vi "create_scan_file.vi"(3 "Scan Type":string(combo)="New Scan", 4 "Scan Name":string, 5 "Scan Directory":string="Peter_ferguson\\test_scans\\Tcal Labview\\") -> (0 "Path Scan":path, 1 "Error Out":errorcluster, 2 "Path Spec":path)   [LabVIEW 2020]
uses:
  <vilib>/Utility/sysdir.llb/System Directory Type.ctl
panel:
  out "output string":string
  in  "Leave File Open (T)":bool=TRUE
  out "Report File Name":path
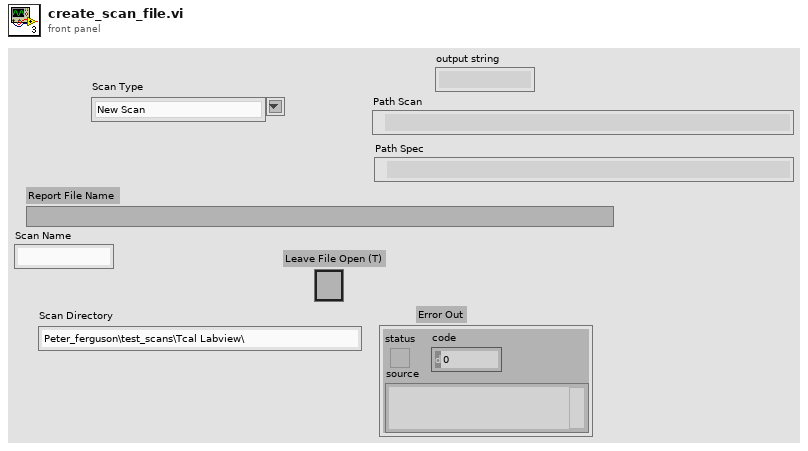
[diagram p1: front panel]
types:
  T1 = typedef "System Directory Type.ctl" = i32
  T2 = enum16{"open", "replace", "create", "open or create", "replace or create", "replace or create with confirmation"}
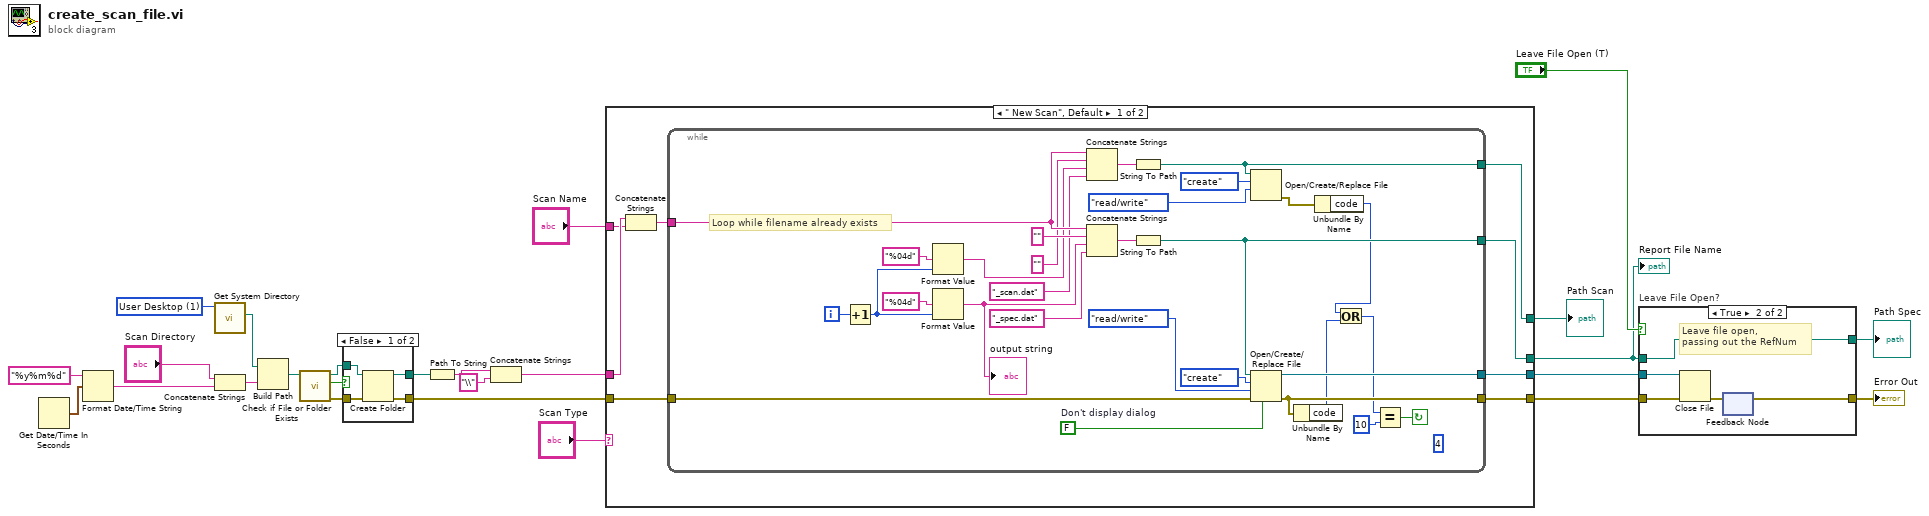
[diagram p0: block diagram]
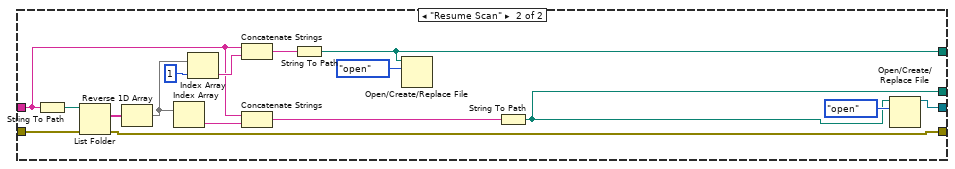
[diagram p2: hidden frame]
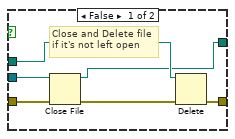
[diagram p4: hidden frame]
diagram:
  w23 = T1 1 items=["User Home"=0, "User Desktop"=1, "User Documents"=2, "User Application Data"=3, "User Preferences"=4, "User Temporary"=5, "Public Documents"=6, "Public Application Data"=7, "Public Preferences"=8, "Public Cache"=13, "System Core Libraries"=9, "System Installed Libraries"=10, "Application Files"=11, "Boot Volume Root"=12] ("system directory type")
  n1 = Get Date/Time In Seconds() -> (seconds since 1Jan1904=w25:timestamp)
  n2 = Format Date/Time String(time format string (%c)="%y%m%d", seconds (now)=w25) -> (date/time string=w20:string)  [unwired: 1 in]
  n3 = call <vilib>:"Get System Directory.vi"("system directory type"=w23) -> ("system directory"=w22:path)  [unwired: 10 in]
  n4 = Concatenate Strings("Scan Directory", w20) -> (w19:string)
  n5 = Build Path(base path=w22, name or relative path=w19) -> (appended path=w10:path)
  n6 = call <vilib>:"Check if File or Folder Exists.vi"("path"=w10) -> ("error out"=w6:errorcluster, "file or folder exists?"=w9:bool, "dup path"=w8:path)  [unwired: 8 in]
  n7 = case shown="False" w9 {
    tunnel: w8 -> [w29 w31]
    tunnel: [w28 w31] -> w7
    tunnel: w6 -> [w27 w30]
    tunnel: [w26 w30] -> w5
    frame False {
      n8 = Create Folder(path (use dialog)=w29, error in=w27) -> (created path=w28:path, error out=w26:errorcluster)  [unwired: 1 in, 1 out]
    }
    frame True {
    }
  }
  n9 = Path To String(path=w7) -> (string=w18:string)
  n10 = Concatenate Strings(w18, "\\") -> (w17:string)
  n11 = case shown="\" New Scan\", Default" "Scan Type" {
    tunnel: w17 -> [w35 w74]
    tunnel: [w39 w78] -> w16
    tunnel: [w38 w83] -> w15
    tunnel: [w37 w72] -> w13
    tunnel: w5 -> [w36 w84]
    tunnel: "Scan Name" -> [w33 _]
    tunnel: [w32 w70] -> w1
    frame " New Scan", Default {
      n12 = Concatenate Strings(w35, w33) -> (w34:string)
      n13 = while {
        tunnel: w36 -> [w58]
        tunnel: [w61] -> w38
        tunnel: [w64] -> w39
        tunnel: [w65] -> w37
        tunnel: w34 -> [w51]
        tunnel: [w44] -> w32
        i -> [w68]
        stop <- w60 continue-if-true
        w63 = FALSE  # Don't display dialog
        (unwired) 4
        # "Loop while filename already exists"
        n14 = Increment(x=w68) -> (x+1=w45:i32)
        n15 = Format Value(format string="%04d", value (0)=w45) -> (output string=w48:string)  [unwired: 1 in]
        n16 = Format Value(format string="%04d", value (0)=w45) -> (output string=w54:string)  [unwired: 1 in]
        "output string" <- w54
        n17 = Concatenate Strings(w51, "", w48, "_scan.dat") -> (w46:string)
        n18 = Concatenate Strings(w51, "", w54, "_spec.dat") -> (w66:string)
        n19 = String To Path(string=w46) -> (path=w44:path)
        n20 = String To Path(string=w66) -> (path=w65:path)
        n21 = Open/Create/Replace File(file path (use dialog)=w44, operation (0:open)=T2."create", access (0:read/write)=enum16{"read/write", "read-only", "write-only"}."read/write") -> (error out=w41:errorcluster)  [unwired: 3 in, 2 out]
        n22 = Open/Create/Replace File(file path (use dialog)=w65, error in=w58, operation (0:open)=T2."create", access (0:read/write)=enum16{"read/write", "read-only", "write-only"}."read/write", disable buffering (F)=w63) -> (refnum out=w64:refnum<file>, error out=w61:errorcluster)  [unwired: 1 in, 1 out]
        n23 = Unbundle By Name(w61) -> ("code"=w43:i32)
        n24 = Unbundle By Name(w41) -> ("code"=w40:i32)
        n25 = Or(x=w40, y=w43) -> (x .or. y?=w42:i32)
        n26 = Equal?(x=w42, y=10) -> (x = y?=w60:bool)
      }
    }
    frame "Resume Scan" {
      n27 = String To Path(string=w74) -> (path=w82:path)
      n28 = List Folder(path=w82, error in=w84) -> (filenames=w81:string[], error out=w83:errorcluster)  [unwired: 2 in, 2 out]
      n29 = Reverse 1D Array(array=w81) -> (reversed array=w76:string[])
      n30 = Index Array(array=w76) -> (element=w75:string)  [unwired: 1 in]
      n31 = Index Array(array=w76, index=1) -> (element=w77:string)
      n32 = Concatenate Strings(w74, w77) -> (w80:string)
      n33 = Concatenate Strings(w74, w75) -> (w73:string)
      n34 = String To Path(string=w80) -> (path=w70:path)
      n35 = Open/Create/Replace File(file path (use dialog)=w70, operation (0:open)=T2."open") -> ()  [unwired: 4 in, 3 out]
      n36 = String To Path(string=w73) -> (path=w72:path)
      n37 = Open/Create/Replace File(file path (use dialog)=w72, operation (0:open)=T2."open") -> (refnum out=w78:refnum<file>)  [unwired: 4 in, 2 out]
    }
  }
  "Report File Name" <- w13
  "Path Scan" <- w1
  n38 = case "Leave File Open?" shown="True" "Leave File Open (T)" {
    tunnel: w16 -> [w90 w95]
    tunnel: w15 -> [w89 w92]
    tunnel: [w87 w93] -> w12
    tunnel: w13 -> [w86 w91]
    tunnel: [w85 w91] -> w11
    frame False {
      # "Close and Delete file\nif it's not left open"
      n39 = Close File(refnum=w90, error in=w89) -> (path=w85:path, error out=w88:errorcluster)
      n40 = Delete(path (use dialog)=w86, error in=w88) -> (error out=w87:errorcluster)  [unwired: 3 in, 2 out]
    }
    frame True {
      # "Leave file open,\npassing out the RefNum"
      n41 = Close File(refnum=w95, error in=w92) -> (error out=w94:errorcluster)  [unwired: 1 out]
      n42 = feedback-in #1(w94) -> ()
      n43 = feedback #1() -> (w93:errorcluster)  [unwired: 1 in]
    }
  }
  "Error Out" <- w12
  "Path Spec" <- w11
